vi "customized_data.vi"() -> ()   [LabVIEW 2015]
uses:
  <vilib>/addons/database/Connection.llb/Conn ObjectReference.ctl
  <vilib>/addons/database/Connection.llb/DB Tools Open Connec (String).vi
  <vilib>/addons/database/Connection.llb/Conn Execute.vi
  <vilib>/addons/database/Recordset.llb/Rec Fetch Recordset Data (R).vi
  <vilib>/addons/database/Recordset.llb/Rec Destroy - Connection.vi
  <vilib>/addons/database/NI_Database_API.lvlib
panel:
  out "connection reference":T1
  out "Data_Table":string[][](array[string])
  out "error Out":errorcluster
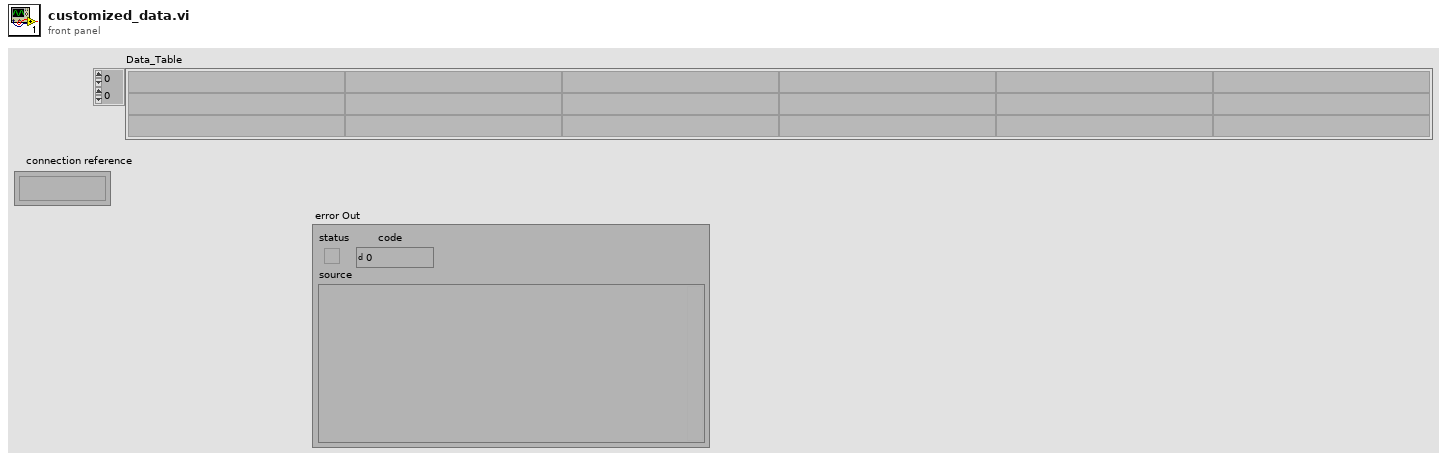
[diagram p1: front panel]
types:
  T1 = typedef "NI_Database_API.lvlib/Conn ObjectReference.ctl" = refnum<k1>
  T2 = typedef "NI_Database_API.lvlib/Rec ObjectReference.ctl" = refnum<k1>
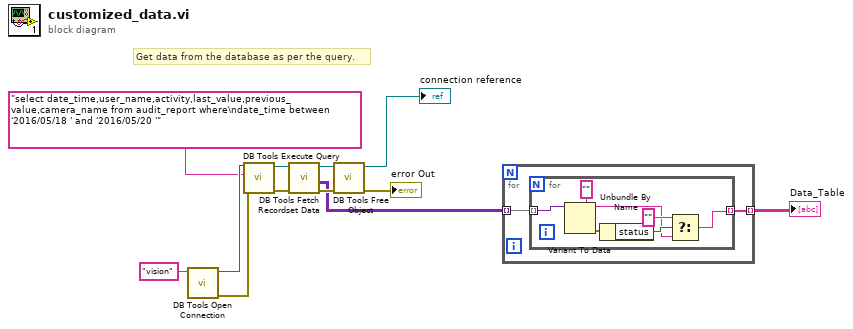
[diagram p0: block diagram]
diagram:
  # "Get data from the database as per the query."
  n1 = call-poly <vilib>:"DB Tools Open Connection.vi"("connection information"="vision" ("SQL query")) -> ("error out"=w1:errorcluster, "connection reference"=w3:T1)  [unwired: 7 in]
  n2 = call-poly <vilib>:"DB Tools Execute Query.vi"("error in (no error)"=w1, "SQL query"="select date_time,user_name,activity,last_value,previous_value,camera_name from audit_report where\ndate_time between '2016/05/18 ' and '2016/05/20 '", "connection reference"=w3) -> ("error out"=w8:errorcluster, "recordset reference"=w9:T2)  [unwired: 5 in]
  n3 = call-poly <vilib>:"DB Tools Fetch Recordset Data.vi"("error in (no error)"=w8, "recordset reference"=w9) -> ("error out"=w10:errorcluster, "recordset data"=w7:variant[][], "recordset reference out"=w11:T2)  [unwired: 3 in]
  n4 = call-poly <vilib>:"DB Tools Free Object.vi"("error in (no error)"=w10, "recordset reference"=w11) -> ("error out"=→"error Out":errorcluster, "connection reference"=→"connection reference":T1)  [unwired: 8 in]
  n5 = for {
    tunnel: w7 -> [w13] mode=indexing
    tunnel: [w14] -> w6 mode=indexing
    n6 = for {
      tunnel: [w15] -> w14 mode=indexing
      tunnel: w13 -> [w20] mode=indexing
      n7 = Variant To Data(type="", Variant=w20) -> (data=w16:string, error out=w19:errorcluster)  [unwired: 1 in]
      n8 = Unbundle By Name(w19) -> ("status"=w18:bool)
      n9 = Select(t="", s=w18, f=w16) -> (s? t:f=w15:string)
    }
  }
  "Data_Table" <- w6
